vi "NeutralOut SetControl.vi"(0 "DeviceReference":T1, 1 "UseTimesync":bool, 7 "error in":errorcluster, 18 "Update Frequency (Hz)":dbl=100.0) -> (20 "DeviceReference Out":T1, 27 "error out":errorcluster)   [LabVIEW 2023]
doc: "Request neutral output of actuator. The applied brake type is determined by the NeutralMode configuration."
uses:
  Users/test.DESKTOP-CORY/Documents/PhoenixProLabVIEWGeneration/CopyDown/DeviceReference.ctl
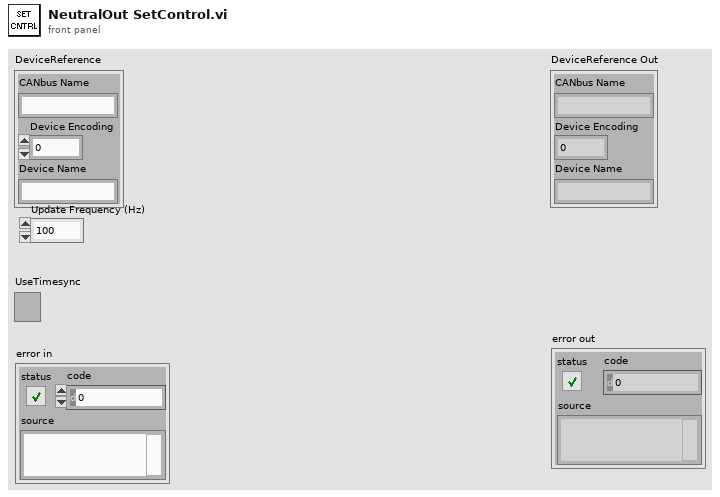
[diagram p1: front panel]
types:
  T1 = typedef "DeviceReference.ctl" = cluster{"CANbus Name":string, "Device Encoding":u32, "Device Name":string}
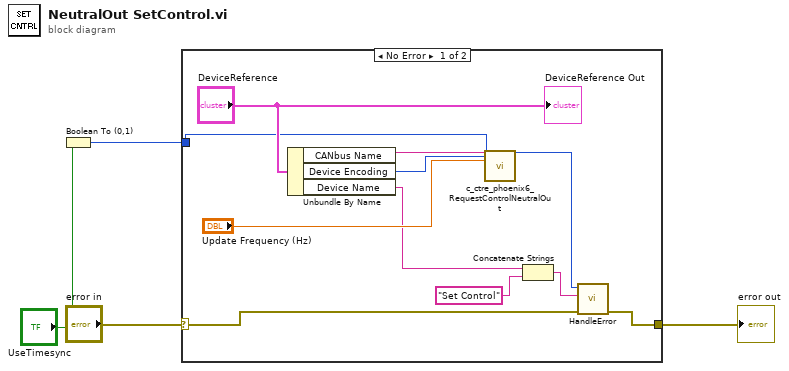
[diagram p0: block diagram]
diagram:
  n1 = Boolean To (0,1)(Boolean="UseTimesync") -> (0, 1=w1:i16)
  n2 = case shown="No Error" "error in" {
    selector: "error in" -> [w10 w16]
    tunnel: [w9 w16] -> w3
    tunnel: w1 -> [w5 _]
    frame No Error {
      n3 = Unbundle By Name("DeviceReference") -> ("CANbus Name"=w14:string, "Device Encoding"=w13:u32, "Device Name"=w8:string)
      n4 = call <vilib>:"c_ctre_phoenix6_RequestControlNeutralOut.vi"("String 2"=w14, "Numeric 2"=w13, "Numeric 3"="Update Frequency (Hz)", 4:w5) -> ("Numeric"=w11:i32)  [unwired: 22 in, 1 out]
      n5 = Concatenate Strings(w8, "Set Control" ("origin")) -> (w6:string)
      n6 = call "HandleError.vi"("error in"=w10, "origin"=w6, "Status"=w11) -> ("error out"=w9:errorcluster)  [unwired: 8 in]
      "DeviceReference Out" <- "DeviceReference"
    }
    frame Error {
    }
  }
  "error out" <- w3
